vi "Get Transfer Identifier.vi"(8 "error in":errorcluster, 9 "label information":cluster{"label number":T1, "sdi":u8} {"label number" format="%.0o"}, 10 "channel number in":u8, 11 "board number in":u8) -> (0 "error out":errorcluster, 2 "new entry created":bool, 3 "Transfer ID out":u32)   [LabVIEW 2020, in "AIM ARINC 429 Hardware API.lvlib"]
uses:
  AIM ARINC 429 Hardware API.lvlib
  Shared/Label.ctl
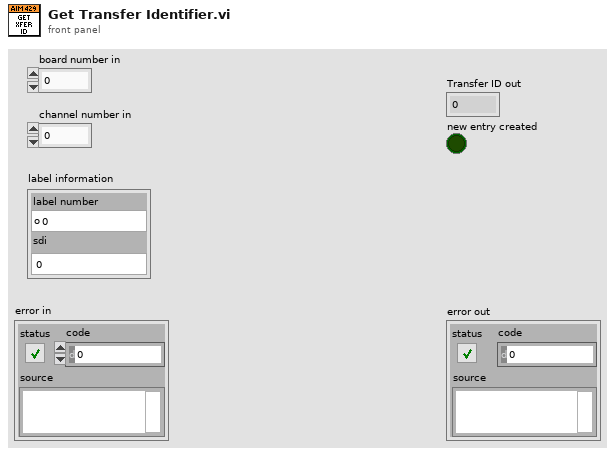
[diagram p1: front panel]
types:
  T1 = typedef "Label.ctl" = u8
  T2 = cluster{"board number in":u8, "channel number in":u8, "label information":cluster{"label number":T1, "sdi":dbl}}
  T3 = map{cluster{"board number in":u8, "channel number in":u8, "label information":cluster{"label number":T1, "sdi":dbl}}, u32}
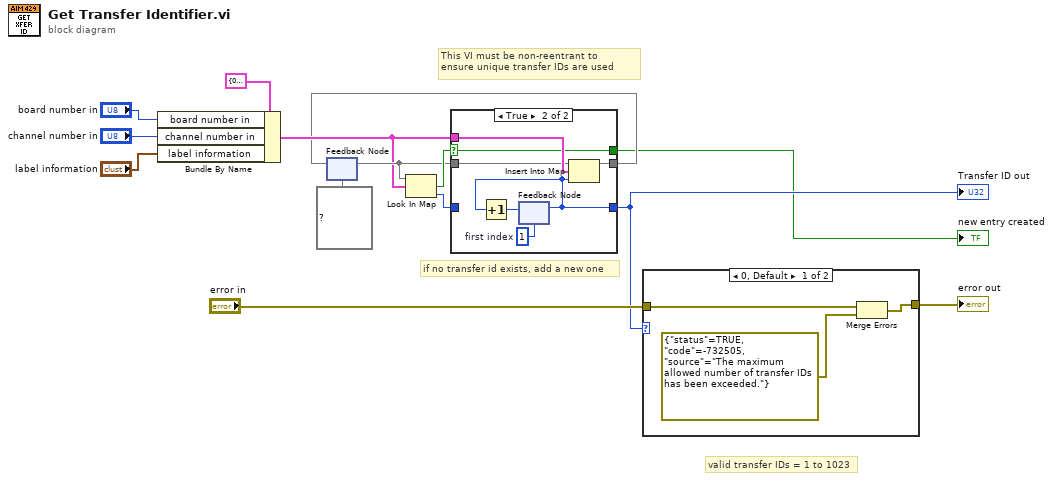
[diagram p0: block diagram]
diagram:
  # "if no transfer id exists, add a new one"
  # "valid transfer IDs = 1 to 1023"
  # "This VI must be non-reentrant to \nensure unique transfer IDs are used"
  n1 = Bundle By Name(cluster=T2 {"board number in"=0, "channel number in"=0, "label information"={"label number"=0, "sdi"=0.0}}, "board number in"="board number in", "channel number in"="channel number in", "label information"="label information") -> (w6:T2)
  n2 = feedback #1(T3 {} ("map")) -> (w7:T3)
  n3 = Look In Map(map=w7, key=w6) -> (key not found?=w9:bool, value=w8:u32)  [unwired: 1 in]
  n4 = case shown="True" w9 {
    selector: w9 -> [w15 w19]
    tunnel: [w17 w18] -> w4
    tunnel: w8 -> [w17 _]
    tunnel: w7 -> [w16 w21]
    tunnel: w6 -> [_ w22]
    tunnel: [w16 w20] -> w5
    tunnel: [w15 w19] -> w3
    frame False {
    }
    frame True {
      w23 = u32 1  # first index
      n5 = feedback #2(w23) -> (w18:u32)
      n6 = Increment(x=w18) -> (x+1=w24:u32)
      n7 = feedback-in #2(w24) -> ()
      n8 = Insert Into Map(map in=w21, key=w22, value=w18) -> (map out=w20:T3)  [unwired: 2 out]
    }
  }
  "Transfer ID out" <- w4
  "new entry created" <- w3
  n9 = feedback-in #1(w5) -> ()
  n10 = case shown="0, Default" w4 {
    tunnel: [w27 w28] -> w14
    tunnel: "error in" -> [w25 w28]
    frame 0, Default {
      n11 = Merge Errors(w25, errorcluster {"status"=TRUE, "code"=-732505, "source"="The maximum allowed number of transfer IDs has been exceeded."} ("error constant")) -> (w27:errorcluster)
    }
    frame 1..1023 {
    }
  }
  "error out" <- w14
